vi "PassFailUUT (SubVI).vi"(8 "error in (no error)":errorcluster, 11 "Table in":refnum<vi>) -> (0 "error out":errorcluster, 2 "Total Pass":u8, 3 "PassFaileUUTresult":bool)   [LabVIEW 2017]
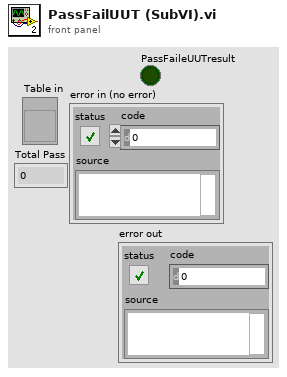
[diagram p1: front panel]
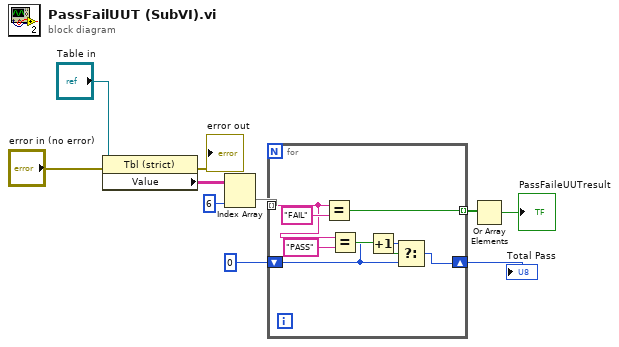
[diagram p0: block diagram]
diagram:
  n1 = property class="Tbl (strict)"(reference="Table in", error in="error in (no error)") -> (error out=→"error out":errorcluster, "Value"=w9:string[][])  [unwired: 1 out]
  n2 = Index Array(array=w9, index (col)=6 ("disabled index (col)")) -> (element=w7:string[])  [unwired: 1 in]
  n3 = for {
    tunnel: w7 -> [w15] mode=indexing
    tunnel: [w17] -> w6 mode=indexing
    shift-right: [w11] -> w1
    shift-left: 0 -> [w13]
    n4 = Equal?(x=w15, y="FAIL") -> (x = y?=w17:bool)
    n5 = Equal?(x=w15, y="PASS") -> (x = y?=w14:bool)
    n6 = Increment(x=w13) -> (x+1=w12:i32)
    n7 = Select(t=w12, s=w14, f=w13) -> (s? t:f=w11:i32)
  }
  "Total Pass" <- w1
  n8 = Or Array Elements(Boolean array=w6) -> (logical OR=→"PassFaileUUTresult":bool)
